vi "Get Custom Device Details.vi"(8 "error in":errorcluster, 11 "Device Reference in":u64 format="%.0x") -> (0 "error out":errorcluster, 3 "Data Reference out":u64=18446744073709551615 format="%.0x", 5 "Custom Device Details":T1)   [LabVIEW 2026, in "NIDMM Engine.lvlib"]
uses:
  NIDMM Engine.lvlib
  <vilib>/NI VeriStand/Custom Device API/Get Item Property (Variant).vi
  <vilib>/NI VeriStand/Custom Device API/Custom Device API.lvlib
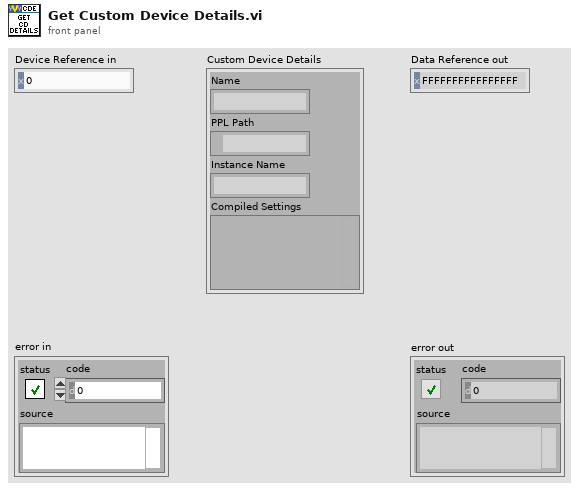
[diagram p1: front panel]
types:
  T1 = cluster{"Name":string, "PPL Path":path, "Instance Name":string, "Compiled Settings":variant}
  T2 = typedef "Custom Device API.lvlib/Custom Device Item Info.ctl" = cluster{"Name":string, "Is Channel":bool, "GUID":string, "Is Waveform":bool}
  T3 = typedef "Custom Device API.lvlib/Custom Device Item Ref.ctl" = u64
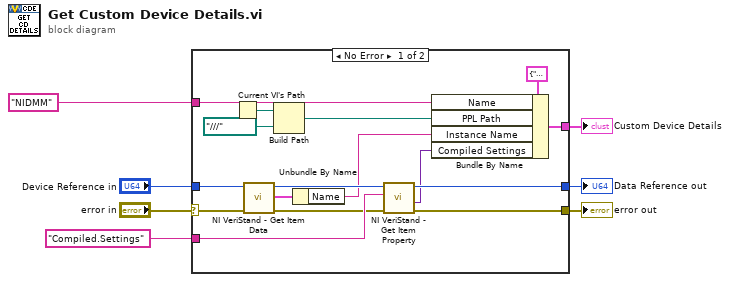
[diagram p0: block diagram]
diagram:
  n1 = case shown="No Error" "error in" {
    selector: "error in" -> [w16 w25]
    tunnel: "Device Reference in" -> [w14 w24]
    tunnel: "Compiled.Settings" ("Property Name") -> [w23 _]
    tunnel: [w22 w25] -> w1
    tunnel: [w21 w24] -> w2
    tunnel: "NIDMM" ("CD.Name") -> [w19 _]
    tunnel: [w18 _] -> w3
    frame No Error {
      n2 = Current VI's Path() -> (path=w10:path)
      n3 = call <vilib>:"NI VeriStand - Get Item Data.vi"("error in (no error)"=w16, "Item Ref in"=w14) -> ("error out"=w15:errorcluster, "Item Info"=w12:T2, "Item Ref out"=w13:T3)  [unwired: 6 in, 1 out]
      n4 = Build Path(base path=w10, name or relative path=path "../../../..") -> (appended path=w8:path)
      n5 = Unbundle By Name(w12) -> ("Name"=w11:string)
      n6 = call-poly <vilib>:"NI VeriStand - Get Item Property.vi"("error in (no error)"=w15, "Property Name"=w23, "Item Ref in"=w13) -> ("error out"=w22:errorcluster, "Value"=w20:variant, "Item Ref out"=w21:T3)  [unwired: 5 in, 1 out]
      n7 = Bundle By Name(cluster=T1 {"Name"="", "PPL Path"=path "", "Instance Name"="", "Compiled Settings"=variant} ("Cluster"), "Name"=w19, "PPL Path"=w8, "Instance Name"=w11, "Compiled Settings"=w20) -> (w18:T1)
    }
    frame Error {
    }
  }
  "Custom Device Details" <- w3
  "Data Reference out" <- w2
  "error out" <- w1
